vi "Start Search.vi"(8 "error in (no error)":errorcluster, 9 "Search Params":T1, 10 "Search":refnum<class "Search.lvclass">, 11 "BetterSearch in":refnum<class "BetterSearch.lvclass">) -> (0 "error out":errorcluster, 3 "BetterSearch out":refnum<class "BetterSearch.lvclass">)   [LabVIEW 2020, in "Better Search.lvlib" / "BetterSearch.lvclass"]
uses:
  BetterSearch.lvclass
  Data Types/Search Params.ctl
  Data Types/Search Type.ctl
  Data Types/Search Scope.ctl
  Data Types/Scope Options.ctl
  Search/Search.lvclass
  BetterSearch.lvclass/BetterSearch.ctl
  Better Search.lvlib
panel:
  # "Exclude"
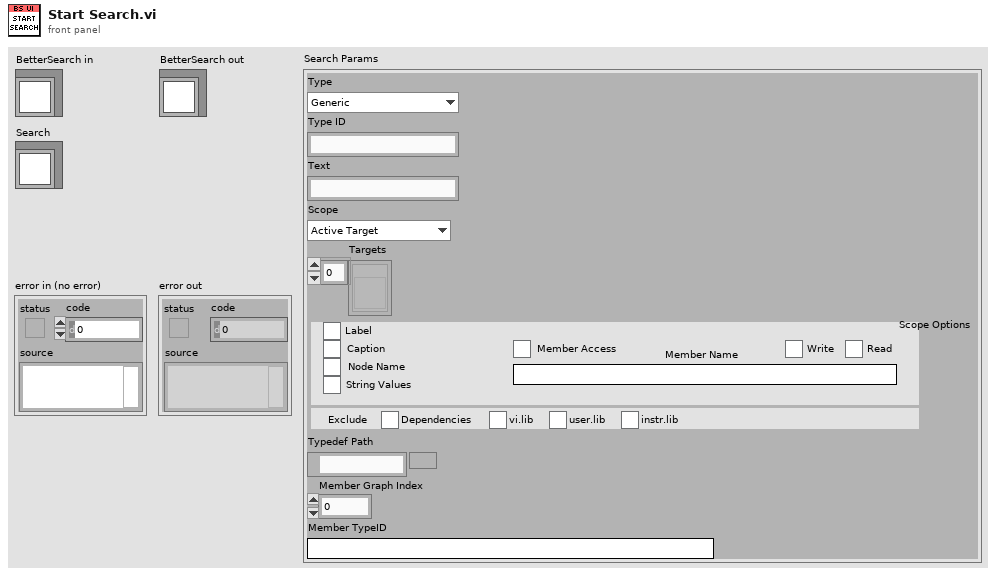
[diagram p1: front panel]
types:
  T1 = typedef "Better Search.lvlib/Search Params.ctl" = cluster{"Type":T2, "Type ID":string, "Text":string, "Scope":T3, "Targets":refnum<vi>[], "Scope Options":T4, "Typedef Path":path, "Member Graph Index":i32, "Member TypeID":string}
  T2 = typedef "Better Search.lvlib/Search Type.ctl" = enum16{"Generic", "Text", "Data Type", "VI", "Node"}
  T3 = typedef "Better Search.lvlib/Search Scope.ctl" = enum16{"Active Target", "Active Project", "Specific Targets", "Active VI", "Active Hierarchy"}
  T4 = typedef "Better Search.lvlib/Scope Options.ctl" = cluster{"Include Labels":bool, "Include Captions":bool, "Include Node Name":bool, "Member Access":bool, "Member Read":bool, "Member Write":bool, "Member Name":string, "String Value":bool, "Dependencies":bool, "vi.lib":bool, "user.lib":bool, "instr.lib":bool}
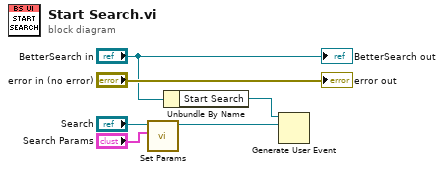
[diagram p0: block diagram]
diagram:
  n1 = call "Set Params.vi"("Search Params"="Search Params", "Search in"="Search") -> ("Search out"=w1:refnum<class "Search.lvclass">)  [unwired: 8 in, 1 out]
  n2 = Unbundle By Name("BetterSearch in") -> ("Start Search"=w4:refnum<user-event>)
  n3 = Generate User Event(user event=w4, event data cluster=w1) -> ()  [unwired: 2 in, 2 out]
  "error out" <- "error in (no error)"
  "BetterSearch out" <- "BetterSearch in"
